vi "Disconnect Channels (Multiple).vi"(8 "error in (no error)":errorcluster, 10 "disconnection list":string, 11 "SLSC Switch in":refnum<class "SLSC Switch.lvclass">) -> (0 "error out":errorcluster, 3 "SLSC Switch out":refnum<class "SLSC Switch.lvclass">)   [LabVIEW 2016, in "SLSC Switch.lvlib" / "SLSC Switch.lvclass"]
doc: "Breaks the connections between channels specified in disconnection list. If no connections exist between channels, SLSC-SWITCH returns an error. In the event of an error, the VI stops at the point in the list where the error occurred."
uses:
  SLSC Switch.lvclass
  SLSC Switch.lvclass/SLSC Switch.ctl
  <vilib>/SLSC/Unflatten Names (String).vi
  slscsl/slscsl.lvclass
  <vilib>/SLSC/SLSC.lvlib
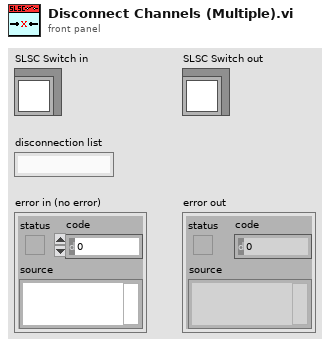
[diagram p1: front panel]
types:
  T1 = typedef "SLSC Switch.lvlib/slscsl.lvclass/SwitchActionsArray.ctl" = T2[]
  T2 = typedef "SLSC Switch.lvlib/slscsl.lvclass/SwitchAction.ctl" = cluster{"index":i32, "RelayAction":T3}
  T3 = typedef "SLSC Switch.lvlib/slscsl.lvclass/RelayAction.ctl" = u32
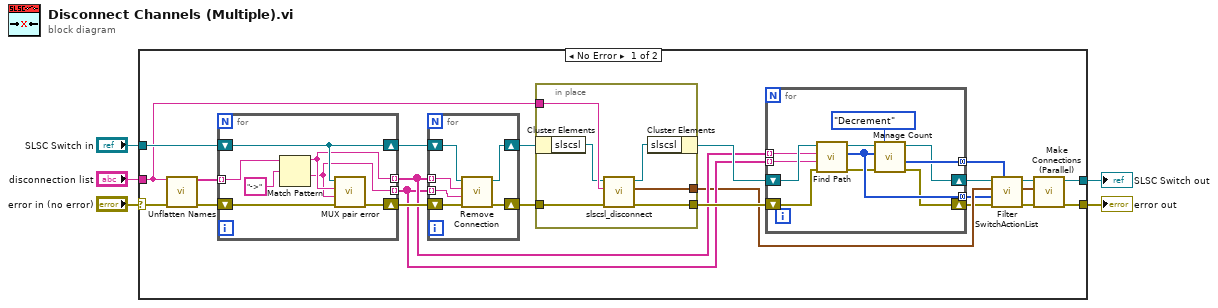
[diagram p0: block diagram]
diagram:
  n1 = case shown="No Error" "error in (no error)" {
    selector: "error in (no error)" -> [w19 w60]
    tunnel: [w23 w60] -> w4
    tunnel: "disconnection list" -> [w21 _]
    tunnel: "SLSC Switch in" -> [w28 w59]
    tunnel: [w24 w59] -> w2
    frame No Error {
      n2 = call-poly <vilib>:"Unflatten Names.vi"("names in"=w21, "error in (no error)"=w19) -> ("names out"=w20:string[], "error out"=w18:errorcluster)  [unwired: 12 in]
      n3 = for {
        tunnel: w20 -> [w45] mode=indexing
        shift-right: [w43] -> w27
        shift-left: w28 -> [w43]
        shift-right: [w40] -> w26
        shift-left: w18 -> [w44]
        tunnel: [w42] -> w13 mode=indexing
        tunnel: [w41] -> w12 mode=indexing
        n4 = Match Pattern(string=w45, regular expression="->") -> (before substring=w42:string, after substring=w41:string)  [unwired: 1 in, 2 out]
        n5 = call "MUX pair error.vi"("error in (no error)"=w44, "channel 2"=w41, "channel 1"=w42, "SLSC Switch in"=w43) -> ("error out"=w40:errorcluster)  [unwired: 7 in]
      }
      n6 = for {
        shift-right: [w51] -> w25
        shift-left: w27 -> [w52]
        shift-right: [w47] -> w22
        shift-left: w26 -> [w50]
        tunnel: w13 -> [w49] mode=indexing
        tunnel: w12 -> [w48] mode=indexing
        n7 = call "Remove Connection.vi"("error in (no error)"=w50, "channel 2"=w48, "channel 1"=w49, "SLSC Switch in"=w52) -> ("error out"=w47:errorcluster, "SLSC Switch out"=w51:refnum<class "SLSC Switch.lvclass">)  [unwired: 6 in]
      }
      n8 = in-place {
        in-place-border: w21 -> [w58]
        in-place-border: w22 -> [w57]
        in-place-border: [w56] -> w15
        in-place-border: [w53] -> w11
        n9 = in-place-cluster #1(w25) -> ("slscsl"=w55:refnum<class "slscsl.lvclass">)
        n10 = call "slscsl_disconnect.vi"("error in (no error)"=w57, "connectionList"=w58, "slscsl in"=w55) -> ("error out"=w56:errorcluster, "SwitchActionsArray"=w53:T1, "slscsl out"=w54:refnum<class "slscsl.lvclass">)  [unwired: 6 in]
        n11 = in-place-cluster #1("slscsl"=w54) -> (w17:refnum<class "SLSC Switch.lvclass">)
      }
      n12 = for {
        tunnel: w13 -> [w37] mode=indexing
        tunnel: w12 -> [w36] mode=indexing
        tunnel: [w34] -> w10 mode=concatenating
        tunnel: [w33] -> w9 mode=concatenating
        shift-right: [w30] -> w8
        shift-left: w17 -> [w39]
        shift-right: [w29] -> w7
        shift-left: w15 -> [w38]
        n13 = call "Find Path.vi"("error in (no error)"=w38, "channel 2"=w36, "channel 1"=w37, "SLSC Switch in"=w39) -> ("error out"=w32:errorcluster, "Relay Indexes"=w33:i32[], "SLSC Switch out"=w31:refnum<class "SLSC Switch.lvclass">)  [unwired: 5 in]
        n14 = call "Manage Count.vi"("Inc/Dec"=enum16{"Increment", "Decrement"}."Decrement", "error in (no error)"=w32, "Relay Indexes"=w33, "SLSC Switch in"=w31) -> ("error out"=w29:errorcluster, "Relay Counts"=w34:i32[], "SLSC Switch out"=w30:refnum<class "SLSC Switch.lvclass">)  [unwired: 5 in]
      }
      n15 = call "Filter SwitchActionList.vi"("Relay Counts"=w10, "error in (no error)"=w7, "Relay Indexes"=w9, "SwitchActionList in"=w11, "SLSC Switch in"=w8) -> ("error out"=w14:errorcluster, "SwitchActionList out"=w6:T1, "SLSC Switch out"=w16:refnum<class "SLSC Switch.lvclass">)  [unwired: 4 in]
      n16 = call "Make Connections (Parallel).vi"("error in (no error)"=w14, "switchActionsArray"=w6, "SLSC Switch in"=w16) -> ("error out"=w23:errorcluster, "SLSC Switch out"=w24:refnum<class "SLSC Switch.lvclass">)  [unwired: 7 in]
    }
    frame Error {
    }
  }
  "error out" <- w4
  "SLSC Switch out" <- w2
